vi "CRYGet Curve Library One Data .vi"(9 "Data Name":string, 11 "Type":enum16{"Curves", "Values", "Results", "WFM"}(ring)) -> (0 "index":i32, 1 "Wave":T3={"Waveform"={"X0"=0.0, "dX"=0.0, "Y"=[]}, "X data"=1, "Y data"=0, "Y axis"=0, "X unit"="s", "Y unit"="", "Y dB ref"=1.0, "display Y"=TRUE, "display X"=FALSE, "Overload?"=FALSE, "Test Info"="", "Step No."=0, "Name"="", "protected"=FALSE, "Sqc history"=[], "Signal Channel ID"=0, "Plot Settings"={"Color"=0, "Interpolation"=0, "Point Style"=0, "Line Style"=0, "Point Color"=0, "Line Width"=0, "Bar Plot Style"=0, "Fill To"=0}, "AutoProtect"=FALSE} {"Y dB ref" format="%.1f"; "Y axis" items=["Log", "Lin"]; "Y data" items=["dB", "Lin"]; "X data" items=["dB", "Lin"]}, 2 "Value":T2={"Name"="", "Curve"=[], "X data"=1, "Y data"=1, "Z data"=1, "X axis"=0, "Y axis"=1, "Z axis"=1, "X unit"="Hz", "Y unit"="", "Z unit"="deg.", "X dB ref"=1.0, "Y dB ref"=1.0, "Z dB ref"=1.0, "single val"=FALSE, "protected"=FALSE, "display X"=TRUE, "display Y"=TRUE, "display Z"=TRUE, "Test Info"="", "Step No."=0, "Plot Settings"={"Color"=0, "Interpolation"=0, "Point Style"=0, "Line Style"=0, "Point Color"=0, "Line Width"=0, "Bar Plot Style"=0, "Fill To"=0}, "AutoProtect"=FALSE} {"Z data" items=["dB", "Lin"]; "X data" items=["dB", "Lin"]; "Y data" items=["dB", "Lin"]; "Z dB ref" format="%.1f"; "Z axis" items=["Log", "Lin"]; "X dB ref" format="%.1f"; "X axis" items=["Log", "Lin"]; "Y axis" items=["Log", "Lin"]; "Y dB ref" format="%.1f"; "Curve"."z" format="%.2f"; "Curve"."y" format="%.2f"; "Curve"."x" format="%.2f"}, 3 "Curve":T2={"Name"="", "Curve"=[], "X data"=1, "Y data"=1, "Z data"=1, "X axis"=0, "Y axis"=1, "Z axis"=1, "X unit"="Hz", "Y unit"="", "Z unit"="deg.", "X dB ref"=1.0, "Y dB ref"=1.0, "Z dB ref"=1.0, "single val"=FALSE, "protected"=FALSE, "display X"=TRUE, "display Y"=TRUE, "display Z"=TRUE, "Test Info"="", "Step No."=0, "Plot Settings"={"Color"=0, "Interpolation"=0, "Point Style"=0, "Line Style"=0, "Point Color"=0, "Line Width"=0, "Bar Plot Style"=0, "Fill To"=0}, "AutoProtect"=FALSE} {"Z data" items=["dB", "Lin"]; "X data" items=["dB", "Lin"]; "Y data" items=["dB", "Lin"]; "Z dB ref" format="%.1f"; "Z axis" items=["Log", "Lin"]; "X dB ref" format="%.1f"; "X axis" items=["Log", "Lin"]; "Y axis" items=["Log", "Lin"]; "Y dB ref" format="%.1f"; "Curve"."z" format="%.2f"; "Curve"."y" format="%.2f"; "Curve"."x" format="%.2f"}, 4 "Result":T1={"Name"="Test for Signal [L]", "Margin"=nan, "unit"="", "Verdict"=FALSE, "Limit"="", "Max/Min"="", "protected"=FALSE, "Step No."=0, "Test Info"="", "AutoProtect"=FALSE} {"Margin" format="%.2f"}, 5 "Result":bool=TRUE, 6 "Step No.":i32)   [LabVIEW 2013]
uses:
  CRYSystem/Typedef Control/CRYWaveform Cluster.ctl
  CRYSystem/Typedef Control/CRYData Cluster.ctl
  CRYSystem/Typedef Control/CRYResult Cluster.ctl
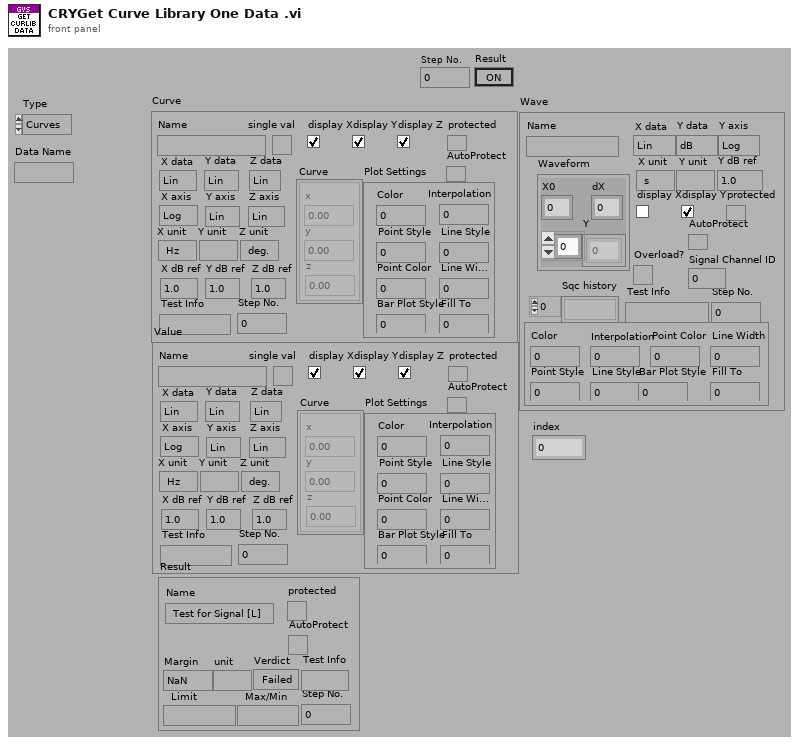
[diagram p1: front panel]
types:
  T1 = typedef "CRYResult Cluster.ctl" = cluster{"Name":string, "Margin":dbl, "unit":string, "Verdict":bool, "Limit":string, "Max/Min":string, "protected":bool, "Step No.":i32, "Test Info":string, "AutoProtect":bool}
  T2 = typedef "CRYData Cluster.ctl" = cluster{"Name":string, "Curve":cluster{"x":dbl, "y":dbl, "z":dbl}[], "X data":u16, "Y data":u16, "Z data":u16, "X axis":u16, "Y axis":u16, "Z axis":u16, "X unit":string, "Y unit":string, "Z unit":string, "X dB ref":dbl, "Y dB ref":dbl, "Z dB ref":dbl, "single val":bool, "protected":bool, "display X":bool, "display Y":bool, "display Z":bool, "Test Info":string, "Step No.":i32, "Plot Settings":cluster{"Color":u32, "Interpolation":u8, "Point Style":u8, "Line Style":u8, "Point Color":u32, "Line Width":u8, "Bar Plot Style":u8, "Fill To":i16}, "AutoProtect":bool}
  T3 = typedef "CRYWaveform Cluster.ctl" = cluster{"Waveform":cluster{"X0":dbl, "dX":dbl, "Y":sgl[]}, "X data":u16, "Y data":u16, "Y axis":u16, "X unit":string, "Y unit":string, "Y dB ref":dbl, "display Y":bool, "display X":bool, "Overload?":bool, "Test Info":string, "Step No.":i32, "Name":string, "protected":bool, "Sqc history":string[], "Signal Channel ID":i32, "Plot Settings":cluster{"Color":u32, "Interpolation":u8, "Point Style":u8, "Line Style":u8, "Point Color":u32, "Line Width":u8, "Bar Plot Style":u8, "Fill To":i16}, "AutoProtect":bool}
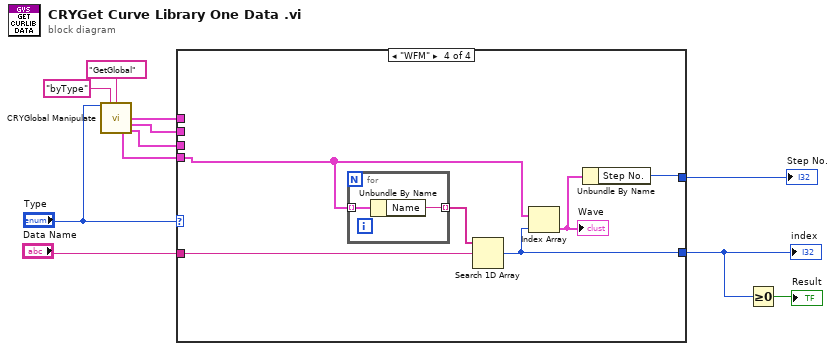
[diagram p0: block diagram]
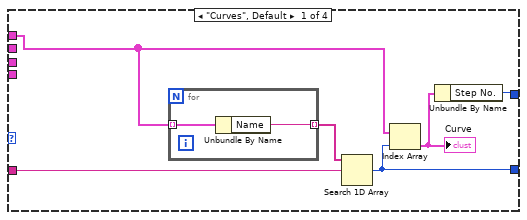
[diagram p2: hidden frame]
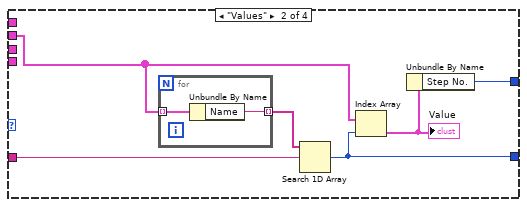
[diagram p3: hidden frame]
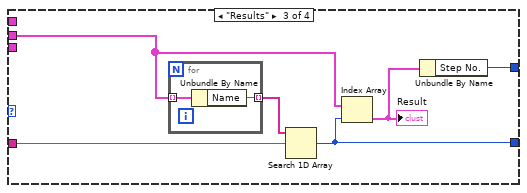
[diagram p4: hidden frame]
diagram:
  n1 = call "CRYGlobal Manipulate.vi"("Type"="Type", "sOption"="byType", "sAction"="GetGlobal") -> ("Curves Out"=w5:T2[], "Values Out"=w4:T2[], "WFM Out"=w2:T3[], "Results Out"=w3:T1[])  [unwired: 6 in, 3 out]
  n2 = case shown="\"WFM\"" "Type" {
    tunnel: "Data Name" -> [w17 w25 w31 w40]
    tunnel: [w15 w24 w32 w39] -> w8
    tunnel: [w13 w21 w29 w37] -> w10
    tunnel: w5 -> [w12 _ _ _]
    tunnel: w4 -> [_ w20 _ _]
    tunnel: w3 -> [_ _ w28 _]
    tunnel: w2 -> [_ _ _ w36]
    frame "Curves", Default {
      n3 = for {
        tunnel: w12 -> [w19] mode=indexing
        tunnel: [w18] -> w16 mode=indexing
        n4 = Unbundle By Name(w19) -> ("Name"=w18:string)
      }
      n5 = Search 1D Array(1D array=w16, element=w17) -> (index of element=w15:i32)  [unwired: 1 in]
      n6 = Index Array(array=w12, index=w15) -> (element=w14:T2)
      "Curve" <- w14
      n7 = Unbundle By Name(w14) -> ("Step No."=w13:i32)
    }
    frame "Values" {
      n8 = for {
        tunnel: w20 -> [w27] mode=indexing
        tunnel: [w26] -> w23 mode=indexing
        n9 = Unbundle By Name(w27) -> ("Name"=w26:string)
      }
      n10 = Search 1D Array(1D array=w23, element=w25) -> (index of element=w24:i32)  [unwired: 1 in]
      n11 = Index Array(array=w20, index=w24) -> (element=w22:T2)
      "Value" <- w22
      n12 = Unbundle By Name(w22) -> ("Step No."=w21:i32)
    }
    frame "Results" {
      n13 = for {
        tunnel: w28 -> [w35] mode=indexing
        tunnel: [w34] -> w33 mode=indexing
        n14 = Unbundle By Name(w35) -> ("Name"=w34:string)
      }
      n15 = Search 1D Array(1D array=w33, element=w31) -> (index of element=w32:i32)  [unwired: 1 in]
      n16 = Index Array(array=w28, index=w32) -> (element=w30:T1)
      "Result" <- w30
      n17 = Unbundle By Name(w30) -> ("Step No."=w29:i32)
    }
    frame "WFM" {
      n18 = for {
        tunnel: w36 -> [w43] mode=indexing
        tunnel: [w42] -> w41 mode=indexing
        n19 = Unbundle By Name(w43) -> ("Name"=w42:string)
      }
      n20 = Search 1D Array(1D array=w41, element=w40) -> (index of element=w39:i32)  [unwired: 1 in]
      n21 = Index Array(array=w36, index=w39) -> (element=w38:T3)
      "Wave" <- w38
      n22 = Unbundle By Name(w38) -> ("Step No."=w37:i32)
    }
  }
  "index" <- w8
  "Step No." <- w10
  n23 = Greater Or Equal To 0?(x=w8) -> (x >= 0?=→"Result":bool)
